vi "get_LCM_from Array.vi"(11 "NoiseFrequency/Hz":i32[](array[numeric])) -> (3 "lcm(x,y)":i64)   [LabVIEW 2018]
uses:
  <vilib>/gmath/NI_Gmath.lvlib
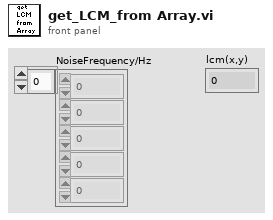
[diagram p1: front panel]
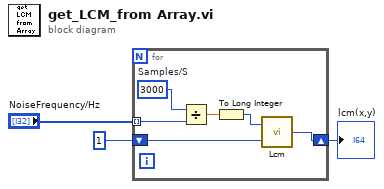
[diagram p0: block diagram]
diagram:
  n1 = for {
    tunnel: "NoiseFrequency/Hz" -> [w7] mode=indexing
    shift-right: [w4] -> w1
    shift-left: 1 -> [w5]
    w9 = 3000  # Samples/S
    n2 = Divide(x=w9, y=w7) -> (x/y=w8:dbl)
    n3 = To Long Integer(number=w8) -> (32bit integer=w6:i32)
    n4 = call <vilib>:"Lcm.vi"("y"=w5, "x"=w6) -> ("lcm(x,y)"=w4:i64)
  }
  "lcm(x,y)" <- w1
